vi "SetXL_CellValues_2D_String.vi"(0 "Refnum Cluster In":T1, 5 "Start":cluster{"Column":i32, "Row":i32}, 9 "data":string[][](array[string]), 11 "error in":errorcluster) -> (4 "Refnum Cluster Out":T1, 15 "error out":errorcluster)   [LabVIEW 2017, in "excel_configuration.lvlib"]
uses:
  excel_configuration.lvlib
  fc58d1ea-0ffd-4866-8301-1bc1faa459e8.vi
  <vilib>/Utility/error.llb/Clear Errors.vi
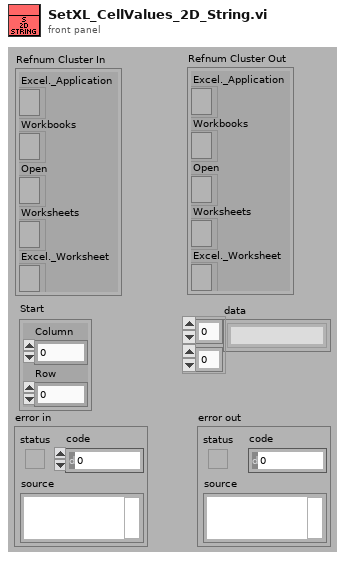
[diagram p1: front panel]
types:
  T1 = cluster{"Excel._Application":refnum<k7>, "Workbooks":refnum<k7>, "Open":refnum<k7>, "Worksheets":refnum<k7>, "Excel._Worksheet":refnum<k7>}
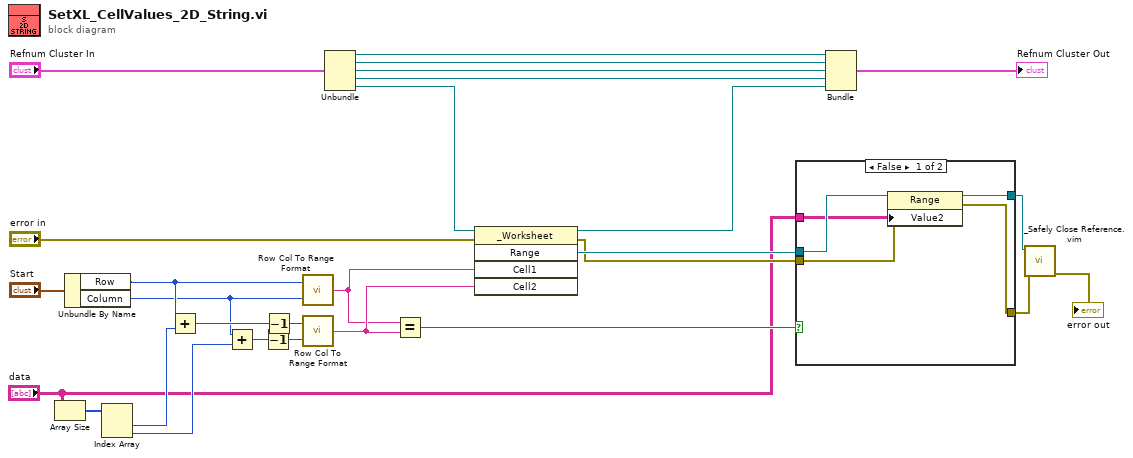
[diagram p0: block diagram]
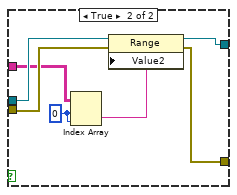
[diagram p2: hidden frame]
diagram:
  n1 = Array Size(array="data") -> (size(s)=w15:i32[])
  n2 = Unbundle By Name("Start") -> ("Row"=w10:i32, "Column"=w9:i32)
  n3 = Index Array(array=w15) -> (element #1=w11:i32, element #2=w12:i32)  [unwired: 2 in]
  n4 = Add(x=w10, y=w11) -> (x+y=w13:i32)
  n5 = Add(x=w9, y=w12) -> (x+y=w14:i32)
  n6 = Decrement(x=w14) -> (x-1=w1:i32)
  n7 = Decrement(x=w13) -> (x-1=w2:i32)
  n8 = call "Row Col To Range Format.vi"("Column"=w9, "Row"=w10) -> ("Output String"=w17:string)
  n9 = call "Row Col To Range Format.vi"("Column"=w1, "Row"=w2) -> ("Output String"=w18:string)
  n10 = Unbundle("Refnum Cluster In") -> ("Excel._Application"=w24:refnum<k7>, "Workbooks"=w25:refnum<k7>, "Open"=w26:refnum<k7>, "Worksheets"=w27:refnum<k7>, "Excel._Worksheet"=w23:refnum<k7>)
  n11 = Equal?(x=w17, y=w18) -> (x = y?=w16:bool)
  n12 = invoke class="_Worksheet" method="Range"(reference=w23, error in="error in", "Cell1"=w17, "Cell2"=w18) -> (reference out=w28:refnum<k7>, error out=w4:errorcluster, "Range"=w6:refnum<k7>)  [unwired: 1 in, 2 out]
  n13 = case shown="False" w16 {
    tunnel: [w30 w39] -> w8
    tunnel: w6 -> [w33 w38]
    tunnel: [w32 w40] -> w5
    tunnel: w4 -> [w31 w37]
    tunnel: "data" -> [w29 w36]
    frame False {
      n14 = property class="Range"(reference=w33, error in=w31, "Value2"=w29) -> (reference out=w32:refnum<k7>, error out=w30:errorcluster)
    }
    frame True {
      w35 = 0 ("index (row)")
      n15 = Index Array(array=w36, index (row)=w35, index (col)=w35) -> (element=w34:string)
      n16 = property class="Range"(reference=w38, error in=w37, "Value2"=w34) -> (reference out=w40:refnum<k7>, error out=w39:errorcluster)
    }
  }
  n17 = Bundle("Excel._Application"=w24, "Workbooks"=w25, "Open"=w26, "Worksheets"=w27, "Excel._Worksheet"=w28) -> (→"Refnum Cluster Out":T1)  [unwired: 1 in]
  n18 = call "_Safely Close Reference.vim"("error in (no error)"=w8, "Automation Refnum in"=w5) -> ("error out"=→"error out":errorcluster)  [unwired: 9 in]
